vi "winningDialog.vi"() -> ()   [LabVIEW 2020]
doc: "Dialog for game winner - simple text and beeping melody. Comments in Polish."
panel:
  in  "Stop":bool
  # "You win !"
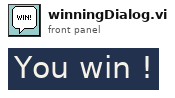
[diagram p1: front panel]
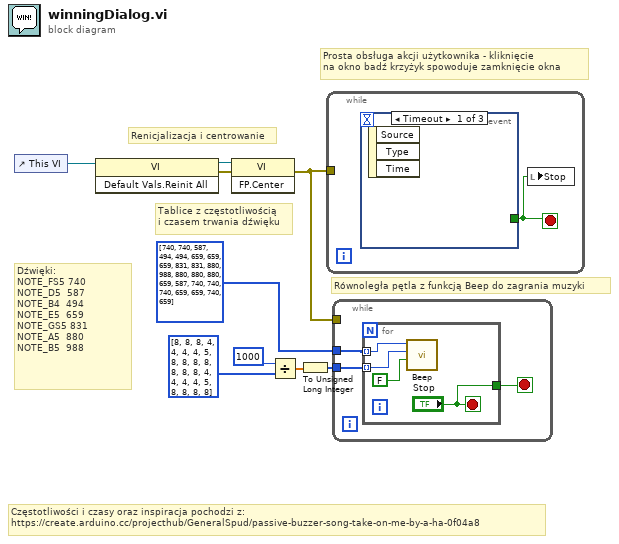
[diagram p0: block diagram]
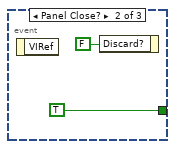
[diagram p2: hidden frame]
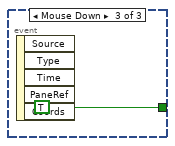
[diagram p3: hidden frame]
diagram:
  # "Tablice z częstotliwością\ni czasem trwania dźwięku"
  # "Równoległa pętla z funkcją Beep do zagrania muzyki"
  # "Prosta obsługa akcji użytkownika - kliknięcie \nna okno badź krzyżyk spowoduje zamknięcie okna"
  # "Renicjalizacja i centrowanie"
  # "Częstotliwości i czasy oraz inspiracja pochodzi z:\nhttps://create.arduino.cc/projecthub/GeneralSpud/passive-buzzer-song-take-on-me-by-a-ha-0f04a8"
  # "Dźwięki:\nNOTE_FS5 740\nNOTE_D5  587\nNOTE_B4  494\nNOTE_E5  659\nNOTE_GS5 831\nNOTE_A5  880\nNOTE_B5  988"
  n1 = control-ref of="This VI"() -> (w6:refnum<vi>)
  n2 = invoke class="VI" method="Default Vals.Reinit All"(reference=w6) -> (reference out=w3:refnum<vi>, error out=w5:errorcluster)  [unwired: 2 in, 1 out]
  n3 = invoke class="VI" method="FP.Center"(reference=w3, error in=w5) -> (error out=w4:errorcluster)  [unwired: 1 in, 2 out]
  n4 = Divide(x=1000 ("duration (msec)"), y=u32[] [8, 8, 8, 4, 4, 4, 4, 5, 8, 8, 8, 8, 8, 8, 8, 4, 4, 4, 4, 5, 8, 8, 8, 8]) -> (x/y=w2:dbl[])
  n5 = To Unsigned Long Integer(number=w2) -> (unsigned 32bit integer=w1:u32[])
  n6 = while {
    tunnel: w4 -> [_]
    stop <- w10 stop-if-true
    n7 = event shown="[0] Timeout" {
      selector: _ -> [_ _ _]
      dyn-events: _ -> [_ _ _]
      timeout: _ -> [_ _ _]
      tunnel: [_ TRUE TRUE] -> w10
      event Timeout {
        n8 = event-data() -> ()  [unwired: 1 in, 3 out]
      }
      event Panel Close? {
        n9 = event-data() -> ()  [unwired: 1 in, 1 out]
        n10 = event-data("Discard?"=FALSE) -> ()  [unwired: 1 in, 1 out]
      }
      event Mouse Down {
        n11 = event-data() -> ()  [unwired: 1 in, 5 out]
      }
    }
    n12 = local write "Stop"(w10) -> ()
  }
  n13 = while {
    tunnel: w1 -> [w16]
    tunnel: u32[] [740, 740, 587, 494, 494, 659, 659, 659, 831, 831, 880, 988, 880, 880, 880, 659, 587, 740, 740, 740, 659, 659, 740, 659] -> [w15]
    tunnel: w4 -> [_]
    stop <- w14 stop-if-true
    n14 = for {
      tunnel: w16 -> [w20] mode=indexing
      tunnel: w15 -> [w19] mode=indexing
      tunnel: ["Stop"] -> w14
      stop <- "Stop" stop-if-true
      n15 = call <vilib>:"Beep.vi"("use system alert? (T)"=FALSE, "duration (msec)"=w20, "frequency (Hz)"=w19) -> ()  [unwired: 9 in]
    }
  }
